vi "Adjust Text Selection.vi"(7 "Remove?":bool, 9 "Length":i32, 10 "Start":i32, 11 "Selection in":T1) -> (3 "Selection out":T1)   [LabVIEW 2023, in "VI Properties Editor.lvlib"]
doc: "Removes HTML bold tags from <B>Value in</B> around <B>Selection in</B>, and modifies the selection to select the same substring as before the removal of the tags."
uses:
  VI Properties Editor.lvlib
  <vilib>/Utility/miscctls.llb/LVSelectionTypeDef.ctl
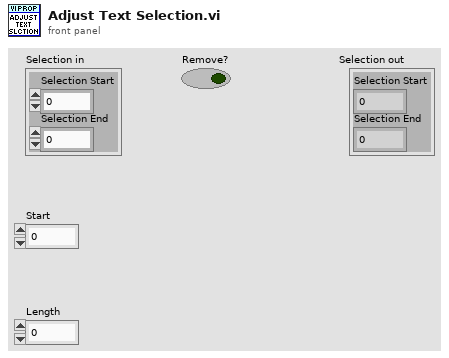
[diagram p1: front panel]
types:
  T1 = typedef "LVSelectionTypeDef.ctl" = cluster{"Selection Start":u32, "Selection End":u32}
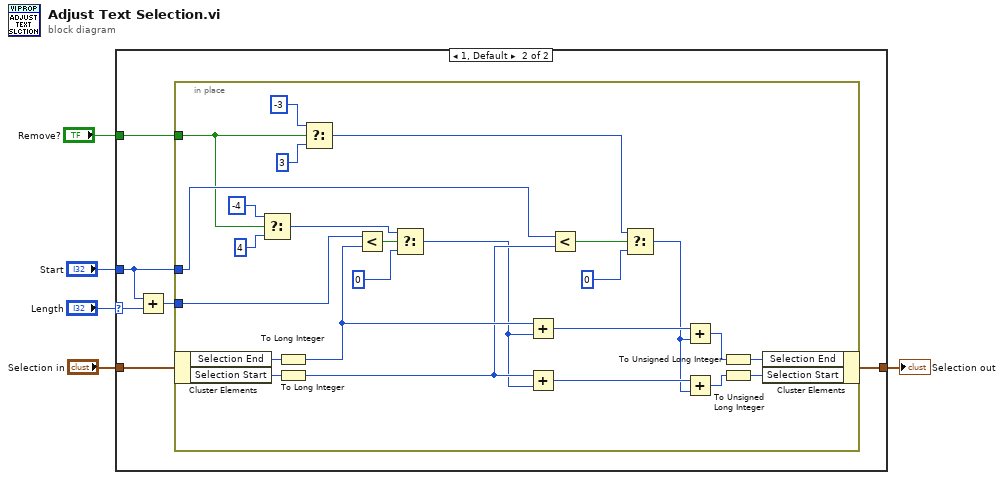
[diagram p0: block diagram]
diagram:
  n1 = case shown="1, Default" "Length" {
    selector: "Length" -> [_ w10]
    tunnel: "Selection in" -> [w6 w12]
    tunnel: [w6 w11] -> w4
    tunnel: "Start" -> [_ w8]
    tunnel: "Remove?" -> [_ w7]
    frame 0 {
    }
    frame 1, Default {
      n2 = Add(x=w8, y=w10) -> (x+y=w9:i32)
      n3 = in-place {
        in-place-border: w9 -> [w28]
        in-place-border: w8 -> [w27]
        in-place-border: w7 -> [w16]
        n4 = in-place-cluster #1(w12) -> ("Selection End"=w30:u32, "Selection Start"=w29:u32)
        n5 = Select(t=-4 ("y"), s=w16, f=4 ("y")) -> (s? t:f=w14:i32)
        n6 = To Long Integer(number=w30) -> (32bit integer=w24:i32)
        n7 = To Long Integer(number=w29) -> (32bit integer=w23:i32)
        n8 = Select(t=-3 ("y"), s=w16, f=3 ("y")) -> (s? t:f=w18:i32)
        n9 = Less?(x=w28, y=w24) -> (x < y?=w37:bool)
        n10 = Select(t=w14, s=w37, f=0 ("y")) -> (s? t:f=w13:i32)
        n11 = Add(x=w24, y=w13) -> (x+y=w36:i32)
        n12 = Add(x=w23, y=w13) -> (x+y=w35:i32)
        n13 = Less?(x=w27, y=w23) -> (x < y?=w34:bool)
        n14 = Select(t=w18, s=w34, f=0 ("y")) -> (s? t:f=w33:i32)
        n15 = Add(x=w36, y=w33) -> (x+y=w32:i32)
        n16 = Add(x=w35, y=w33) -> (x+y=w31:i32)
        n17 = To Unsigned Long Integer(number=w32) -> (unsigned 32bit integer=w25:u32)
        n18 = To Unsigned Long Integer(number=w31) -> (unsigned 32bit integer=w26:u32)
        n19 = in-place-cluster #1("Selection End"=w25, "Selection Start"=w26) -> (w11:T1)
      }
    }
  }
  "Selection out" <- w4
